vi "unit convert.vi"(11 "unit string":string) -> (3 "unit string out":string)   [LabVIEW 2015, in "AguaClara Library.lvlib"]
uses:
  AguaClara Library.lvlib
panel:
  in  "volume":string[](array[string])=["gal", "ml", "l"]
  in  "time":string[](array[string])=["d", "min", "hr"]
  in  "Length":string[](array[string])=["in", "cm", "mm"]
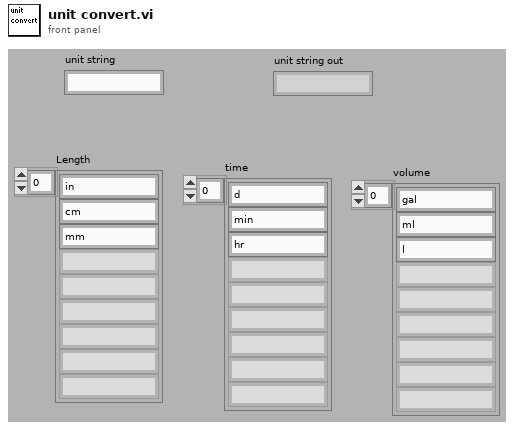
[diagram p1: front panel]
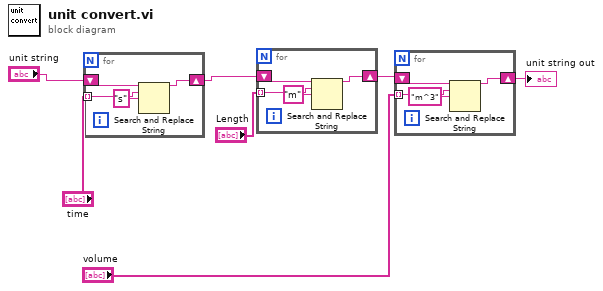
[diagram p0: block diagram]
diagram:
  n1 = for {
    tunnel: "time" -> [w9] mode=indexing
    shift-right: [w10] -> w2
    shift-left: "unit string" -> [w11]
    n2 = Search and Replace String(input string=w11, search string=w9, replace string="s" ("replace string (\"\")")) -> (result string=w10:string)  [unwired: 5 in, 3 out]
  }
  n3 = for {
    tunnel: "Length" -> [w13] mode=indexing
    shift-right: [w14] -> w1
    shift-left: w2 -> [w15]
    n4 = Search and Replace String(input string=w15, search string=w13, replace string="m" ("replace string (\"\")")) -> (result string=w14:string)  [unwired: 5 in, 3 out]
  }
  n5 = for {
    tunnel: "volume" -> [w17] mode=indexing
    shift-right: [w18] -> w4
    shift-left: w1 -> [w19]
    n6 = Search and Replace String(input string=w19, search string=w17, replace string="m^3" ("replace string (\"\")")) -> (result string=w18:string)  [unwired: 5 in, 3 out]
  }
  "unit string out" <- w4
